vi "VI Pop Up_Calgas-Popup.vi"(10 "Zentrieren":bool=TRUE, 11 "VI Referenz":refnum<vi>) -> ()   [LabVIEW 2020, in "allgemeine Sub-VIs.lvlib"]
uses:
  allgemeine Sub-VIs.lvlib
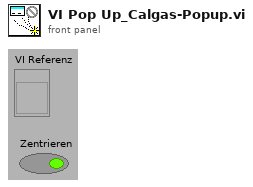
[diagram p1: front panel]
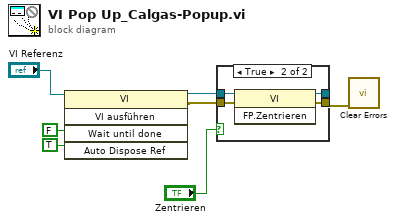
[diagram p0: block diagram]
diagram:
  n1 = invoke class="VI" method="VI ausführen"(reference="VI Referenz", "Wait until done"=FALSE ("Warten bis beendet"), "Auto Dispose Ref"=TRUE ("Referenz automatisch schließen")) -> (reference out=w3:refnum<vi>, error out=w2:errorcluster)  [unwired: 2 in, 3 out]
  n2 = case shown="True" "Zentrieren" {
    tunnel: w3 -> [w9 w13]
    tunnel: w2 -> [w8 w12]
    tunnel: [w8 w11] -> w1
    tunnel: [w9 w10] -> _
    frame False {
    }
    frame True {
      n3 = invoke class="VI" method="FP.Zentrieren"(reference=w13, error in=w12) -> (reference out=w10:refnum<vi>, error out=w11:errorcluster)  [unwired: 1 in, 1 out]
    }
  }
  n4 = call <vilib>:"Clear Errors.vi"("error in (no error)"=w1) -> ()  [unwired: 5 in, 2 out]
